vi "test_in_creating_lookuptables.vi"() -> (0 "Init Data Out":i16[](array[numeric]))   [LabVIEW 2009]
panel:
  # "For Initialization VI requirements and help, please read directions located on Block Diagram."
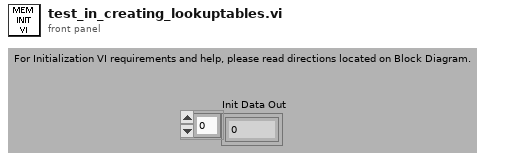
[diagram p1: front panel]
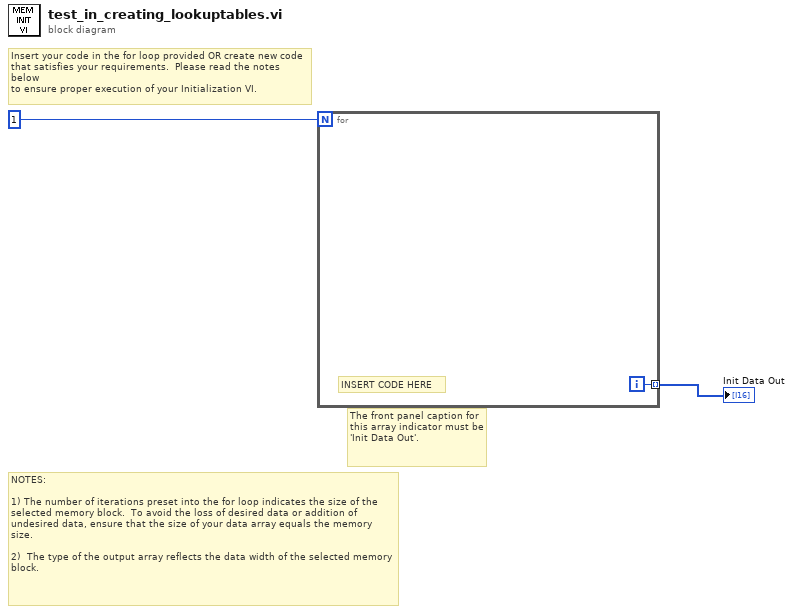
[diagram p0: block diagram]
diagram:
  # "The front panel caption for this array indicator must be 'Init Data Out'."
  # "NOTES:\n\n1) The number of iterations preset into the for loop indicates the size of the selected memory block.  To avoid the loss of desired data or addition of undesired data, ensure that the size of your data array equals the memory size.\n\n2)  The type of the output array reflects the data width of the selected memory block."
  # "Insert your code in the for loop provided OR create new code\nthat satisfies your requirements.  Please read the notes below\nto ensure proper execution of your Initialization VI."
  n1 = for {
    N: u32 1 -> [_]
    tunnel: [w3] -> w1 mode=indexing
    i -> [w3]
    # "INSERT CODE HERE"
  }
  "Init Data Out" <- w1
